vi "Example Callback - Position Callback.vi"(4 "Positiion":refnum<user-event>, 5 "Event Data":cluster{"sender":refnum<k24>, "position":u8}, 6 "Control Ref":refnum<k24>, 7 "Event Common Data":T1) -> ()   [LabVIEW 2013]
uses:
  C:/tf/play/labview/Tinkerforge.dll
  Tinkerforge.dll
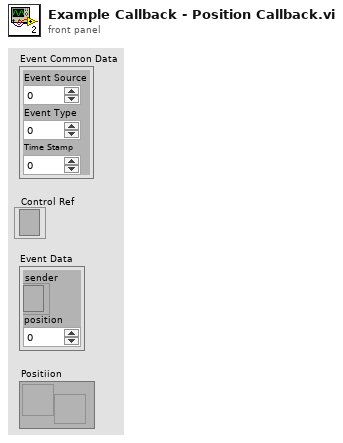
[diagram p1: front panel]
types:
  T1 = cluster{"Event Source":i32, "Event Type":u32, "Time Stamp":u32}
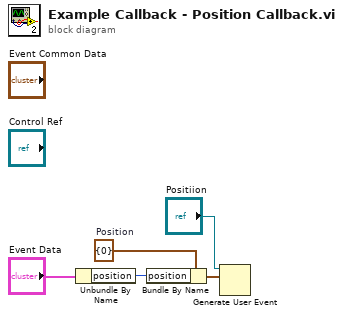
[diagram p0: block diagram]
diagram:
  w2 = cluster{"position":u8} {"position"=0}  # Position
  n1 = Unbundle By Name("Event Data") -> ("position"=w5:u8)
  n2 = Bundle By Name(cluster=w2, "position"=w5) -> (w1:cluster{"position":u8})
  n3 = Generate User Event(user event="Positiion", event data cluster=w1) -> ()  [unwired: 2 in, 2 out]
